vi "rqcBob Channel Test - 2 SPD (Low Level Example).vi"() -> ()   [LabVIEW 2019]
uses:
  FPGA/rqcBob/Custom Controls/Pulse Train/rqcBob Pulse Train Config.ctl
  FPGA/rqcBob/Custom Controls/Pulse Train/rqcBob Pulse Train.Generation Mode.ctl
  FPGA/rqcBob/Custom Controls/Pulse Train/rqcBob Pulse Train.First Pulse Delay Mode.ctl
  FPGA/rqcBob/Custom Controls/rqcBob Modulator Config.ctl
  FPGA/rqcBob/Custom Controls/rqcBob Window Config.ctl
  Shared/Shared FPGA Lib/Shared Logic/Custom Controls/rqc Random Generator.parameters.ctl
  Shared/Shared FPGA Lib/Shared Logic/Custom Controls/rqc Random Generator.value type.ctl
  FPGA/rqcBob/Custom Controls/rqcBob Trigger Type.ctl
  <vilib>/FPGAPlugInAG/PCIe-7820R/niLvFpga_Open_PCIe-7820R.vi
  <vilib>/rvi/interface/common/dynamic/niFpgaDynamicAddResources.vi
  Low Level API/Configuration/Photon Detector/Detection FIFOs config/rqcBob Configure PD Detect FIFO (2PD).vi
  Low Level API/Read/Read PD Detection FIFO/rqcBob Read PD Detection FIFO (1PD PD1).vi
  Low Level API/Read/Read PD Detection FIFO/rqcBob Read PD Detection FIFO (1PD PD2).vi
  <vilib>/FPGAPlugInAG/Dynamic/niLvFpga_Close_Dynamic.vi
  <vilib>/rvi/interface/nirviOpenFPGA/nirviOpenFPGA.xnode
  FPGA Bitfiles/rqcBob (FPGA) 7820  (MB_SPARTAN7) v 4.0.0.lvbitx.lvbitx
  <vilib>/rvi/interface/nirviCloseFPGA/nirviCloseFPGA.xnode
  <vilib>/Analysis/NI_AALPro.lvlib
panel:
  in  "Tab Control":T1(tab)
  in  "train.configuration":T2={"period"=0, "num of pulses"=0, "mode"=enum."train sequence.single", "num of trains"=0, "first pulse delay mode"=enum."every train", "first pulse delay"=55} caption="Pulsed laser configuration"
  in  "modulator.config":T5 caption="Phase modulation"
  in  "window.config":T6 caption="Registration of detector clicks"
  in  "rndGen.parameters":T7={"value type"=enum."constant", "constant"=0, "num of levels"=4, "levels values"=[0, 0, 0, 0]} caption="Phase modulation value" {"num of levels" min=4 max=4 step=1}
  out "Parameters Check Msg":string="Selected parameter combination\nmay lead to inappropriate measurement results"
  in  "Blank Button":bool
  out "SPD.max meas length":u32 caption="SPD max measurement length (in units of 5ns)"
  in  "modulator.clock delay":fxp<+,4,4> caption="PM Clock Delay (0-7) (in units of 40ns)"
  out "2-nd Detector Clicks":T9(graph)
  out "1-st Detector Clicks":T9(graph)
  out "Done":bool=TRUE
  in  "stop":bool
  in  "train.software trigger":bool
  # "Constant"
  # "Random"
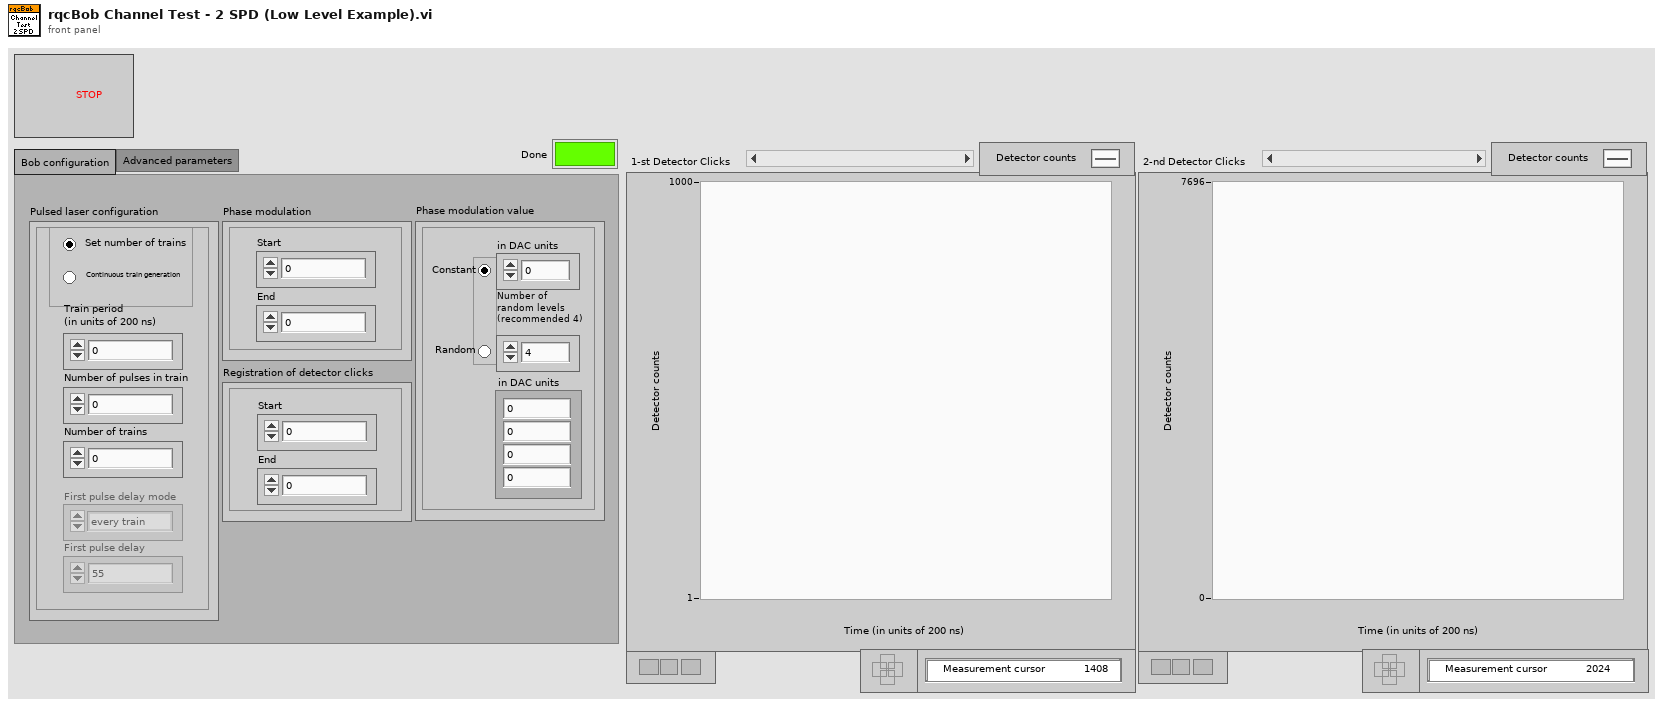
[diagram p1: front panel]
types:
  T1 = enum32{"Bob configuration", "Advanced parameters"}
  T2 = typedef "rqcBob Pulse Train Config.ctl" = cluster{"period":u16, "num of pulses":u16, "mode":T3, "num of trains":u16, "first pulse delay mode":T4, "first pulse delay":u16}
  T3 = typedef "rqcBob Pulse Train.Generation Mode.ctl" = enum32{"single train", "train sequence.single", "train sequence.wait for trigger", "continuous"}
  T4 = typedef "rqcBob Pulse Train.First Pulse Delay Mode.ctl" = enum8{"none", "every train", "first train"}
  T5 = typedef "rqcBob Modulator Config.ctl" = cluster{"modulator.start":u16, "modulator.stop":u16}
  T6 = typedef "rqcBob Window Config.ctl" = cluster{"window.open":u16, "window.close":u16}
  T7 = typedef "rqc Random Generator.parameters.ctl" = cluster{"value type":T8, "constant":u16, "num of levels":u16, "levels values":u16[]}
  T8 = typedef "rqc Random Generator.value type.ctl" = enum32{"random value", "constant"}
  T9 = cluster{"X Values":dbl[], "Histogram: h(x)":i32[]}
  T10 = typedef "rqcBob Trigger Type.ctl" = enum16{"software", "immediate", "DIO"}
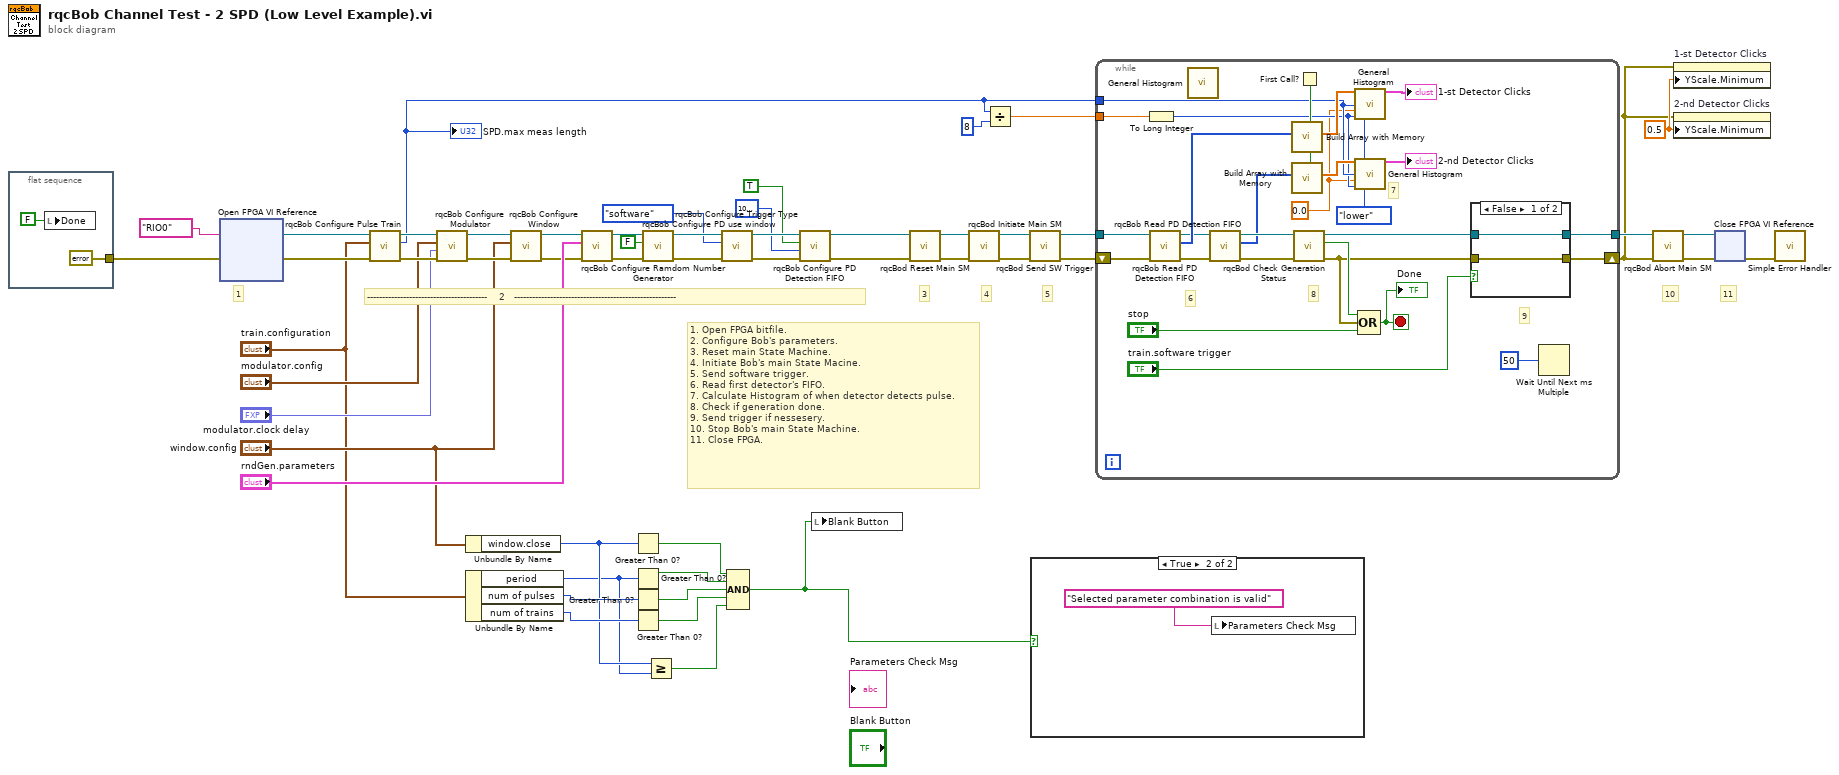
[diagram p0: block diagram]
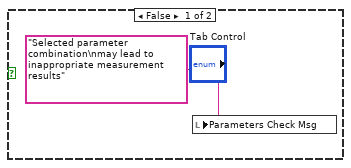
[diagram p2: hidden frame]
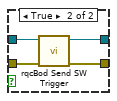
[diagram p3: hidden frame]
diagram:
  w5 = 0.5 ("Y Scale.Range:Minimum")
  # "1. Open FPGA bitfile.\n2. Configure Bob's parameters.\n3. Reset main State Machine.\n4. Initiate Bob's main State Macine.\n5. Send software trigger.\n6. Read first detector's FIFO.\n7. Calculate Histogram of when detector detects pulse.\n8. Check if generation done.\n9. Send trigger if nessesery.\n10. Stop Bob's main State Machine.\n11. Close FPGA."
  # "1"
  # "11"
  # "10"
  # "5"
  # "4"
  # "3"
  # "----------------------------------------    2   ------------------------------------------------------"
  n1 = flat-sequence {
    tunnel: [errorcluster {"status"=FALSE, "code"=0, "source"=""} ("error in")] -> w30
    frame #0 {
      n2 = local write "Done"(FALSE ("Done")) -> ()
    }
  }
  n3 = xnode "Open FPGA VI Reference"("error in"=w30, "resource name"=tag "RIO0") -> ("FPGA VI Reference Out"=w27:refnum<k20>, "error out"=w26:errorcluster)
  n4 = call "rqcBob Configure Pulse Train.vi"("error in"=w26, "train.configuration"="train.configuration", "FPGA reference in"=w27) -> ("error out"=w50:errorcluster, "SPD meas length"=w3:u32, "FPGA reference out"=w51:refnum<k20>)  [unwired: 6 in]
  "SPD.max meas length" <- w3
  n5 = call "rqcBob Configure Modulator.vi"("error in"=w50, "modulator.clock delay"="modulator.clock delay", "modulator.config"="modulator.config", "FPGA reference in"=w51) -> ("error out"=w47:errorcluster, "FPGA reference out"=w48:refnum<k20>)  [unwired: 6 in]
  n6 = Unbundle By Name("window.config") -> ("window.close"=w11:u16)
  n7 = Unbundle By Name("train.configuration") -> ("period"=w10:u16, "num of pulses"=w17:u16, "num of trains"=w16:u16)
  n8 = call "rqcBob Configure Window.vi"("error in"=w47, "window.config"="window.config", "FPGA reference in"=w48) -> ("error out"=w44:errorcluster, "FPGA reference out"=w45:refnum<k20>)  [unwired: 7 in]
  n9 = call "rqcBob Configure Ramdom Number Generator.vi"("error in"=w44, "rqcBob rndGen.parameters"="rndGen.parameters", "FPGA reference in"=w45) -> ("error out"=w43:errorcluster, "FPGA reference out"=w42:refnum<k20>)  [unwired: 7 in]
  n10 = Greater Than 0?(x=w11) -> (x > 0?=w12:bool)
  n11 = Greater Than 0?(x=w10) -> (x > 0?=w13:bool)
  n12 = Greater Than 0?(x=w17) -> (x > 0?=w15:bool)
  n13 = Greater Than 0?(x=w16) -> (x > 0?=w14:bool)
  n14 = call "rqcBob Configure PD use window.vi"("error in"=w43, "PD.use window"=FALSE ("SPD.use detector window"), "FPGA reference in"=w42) -> ("error out"=w40:errorcluster, "FPGA reference out"=w41:refnum<k20>)  [unwired: 7 in]
  n15 = Greater Or Equal?(x=w11, y=w10) -> (x >= y?=w9:bool)
  n16 = call "rqcBob Configure Trigger Type.vi"("error in"=w40, "rqcBob Trigger Type"=rqcBob_Trigger_Type."software", "FPGA reference in"=w41) -> ("error out"=w22:errorcluster, "FPGA reference out"=w24:refnum<k20>)  [unwired: 7 in]
  n17 = Compound Arithmetic op=AND(w12, w13, w15, w14, w9) -> (w8:bool)
  n18 = call-poly "rqcBob Configure PD Detection FIFO.vi"("error in"=w22, "PD.detect fifo depth"=u32 1000000 ("SPD.detect fifo depth"), "PD.detect fifo write enable"=TRUE ("SPD.detect fifo write enable"), "FPGA reference in"=w24) -> ("error out"=w21:errorcluster, "FPGA reference out"=w23:refnum<k20>)  [unwired: 6 in]
  n19 = local write "Blank Button"(w8) -> ()
  n20 = call "rqcBod Reset Main SM.vi"("error in"=w21, "FPGA reference in"=w23) -> ("error out"=w37:errorcluster, "FPGA reference out"=w38:refnum<k20>)  [unwired: 8 in]
  n21 = call "rqcBod Initiate Main SM.vi"("error in"=w37, "FPGA reference in"=w38) -> ("error out"=w35:errorcluster, "FPGA reference out"=w36:refnum<k20>)  [unwired: 8 in]
  n22 = Divide(x=w3, y=u32 8) -> (x/y=w1:dbl)
  n23 = call "rqcBod Send SW Trigger.vi"("error in"=w35, "FPGA reference in"=w36) -> ("error out"=w33:errorcluster, "FPGA reference out"=w34:refnum<k20>)  [unwired: 8 in]
  n24 = case shown="True" w8 {
    frame False {
      n25 = local write "Parameters Check Msg"("Selected parameter combination\nmay lead to inappropriate measurement results") -> ()
    }
    frame True {
      n26 = local write "Parameters Check Msg"("Selected parameter combination is valid") -> ()
    }
  }
  n27 = while {
    tunnel: w34 -> [w74]
    shift-right: [w79] -> w4
    shift-left: w33 -> [w72]
    tunnel: w3 -> [w61]
    tunnel: [w78] -> w18
    tunnel: w1 -> [w60]
    stop <- w76 stop-if-true
    w57 = enum32{"lower", "upper"}."lower" ("inclusion")
    w58 = 0.0 ("min")
    # "7"
    # "9"
    # "8"
    # "6"
    n28 = To Long Integer(number=w60) -> (32bit integer=w59:i32)
    n29 = call-poly "rqcBob Read PD Detection FIFO.vi"("error in"=w72, "FPGA reference in"=w74) -> ("error out"=w64:errorcluster, "Data"=w73:u32[], "FPGA reference out"=w66:refnum<k20>)  [unwired: 6 in, 1 out]
    n30 = call <vilib>:"General Histogram.vi"() -> ()  [unwired: 11 in, 5 out]
    n31 = call-poly "rqcBob Read PD Detection FIFO.vi"("error in"=w64, "FPGA reference in"=w66) -> ("error out"=w63:errorcluster, "Data"=w62:u32[], "FPGA reference out"=w65:refnum<k20>)  [unwired: 6 in, 1 out]
    n32 = call "rqcBod Check Generation Status.vi"("error in"=w63, "FPGA reference in"=w65) -> ("error out"=w80:errorcluster, "generation.done"=w82:bool, "FPGA reference out"=w81:refnum<k20>)  [unwired: 7 in]
    n33 = First Call?() -> (First Call?: T/F=w69:bool)
    n34 = call "Build Array with Memory.vi"("reset"=w69, "new array"=w73) -> ("appended array"=w71:dbl[])  [unwired: 9 in]
    n35 = call "Build Array with Memory.vi"("reset"=w69, "new array"=w62) -> ("appended array"=w67:dbl[])  [unwired: 9 in]
    n36 = call <vilib>:"General Histogram.vi"("X"=w71, "max"=w61, "min"=w58, "# bins"=w59, "inclusion"=w57) -> ("Histogram Graph"=→"1-st Detector Clicks":T9)  [unwired: 6 in, 4 out]
    n37 = call <vilib>:"General Histogram.vi"("X"=w67, "max"=w61, "min"=w58, "# bins"=w59, "inclusion"=w57) -> ("Histogram Graph"=→"2-nd Detector Clicks":T9)  [unwired: 6 in, 4 out]
    n38 = Compound Arithmetic op=OR(w82, w80, "stop") -> (w76:bool)
    "Done" <- w76
    n39 = case shown="False" "train.software trigger" {
      tunnel: w81 -> [w85 w89]
      tunnel: w80 -> [w84 w88]
      tunnel: [w85 w87] -> w78
      tunnel: [w84 w86] -> w79
      frame False {
      }
      frame True {
        n40 = call "rqcBod Send SW Trigger.vi"("error in"=w88, "FPGA reference in"=w89) -> ("error out"=w86:errorcluster, "FPGA reference out"=w87:refnum<k20>)  [unwired: 8 in]
      }
    }
    n41 = Wait Until Next ms Multiple(millisecond multiple=u32 50) -> ()  [unwired: 1 out]
  }
  n42 = call "rqcBod Abort Main SM.vi"("error in"=w4, "FPGA reference in"=w18) -> ("error out"=w31:errorcluster, "FPGA reference out"=w32:refnum<k20>)  [unwired: 8 in]
  n43 = property on="1-st Detector Clicks" class="XYGraph (strict)"(error in=w4, "YScale.Minimum"=w5) -> ()  [unwired: 1 in, 2 out]
  n44 = property on="2-nd Detector Clicks" class="XYGraph (strict)"(error in=w4, "YScale.Minimum"=w5) -> ()  [unwired: 1 in, 2 out]
  n45 = xnode "Close FPGA VI Reference"("FPGA VI Reference In"=w32, "error in"=w31) -> ("error out"=w29:errorcluster)
  n46 = call <vilib>:"Simple Error Handler.vi"("error in (no error)"=w29) -> ()  [unwired: 4 in, 5 out]
